vi "asdk Send.vi"(8 "error in (no error)":errorcluster, 10 "value":dbl[](array[numeric]), 11 "pDm":u32) -> (0 "error out":errorcluster, 3 "pDm out":u32)   [LabVIEW 2019, in "ASDK.lvlib"]
doc: "ASDK_API COMPL_STAT asdkSend( asdkDM *pDm, const Scalar *value );"
uses:
  <userlib>/asdk.lib/ASDK.lvlib
  ASDK.dll
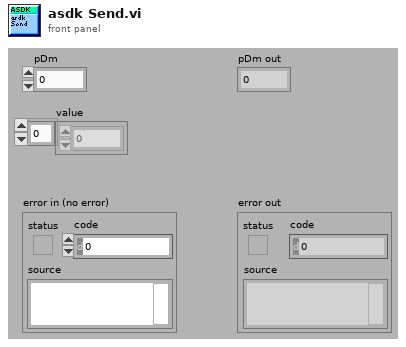
[diagram p1: front panel]
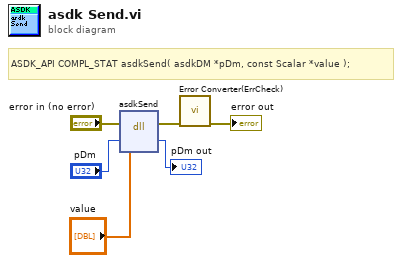
[diagram p0: block diagram]
diagram:
  # "ASDK_API COMPL_STAT asdkSend( asdkDM *pDm, const Scalar *value );"
  n1 = dll-call lib="ASDK.*" fn="asdkSend"(error in="error in (no error)", "pDm"="pDm", "value"="value") -> (error out=w3:errorcluster, "pDm"=→"pDm out":u32)  [unwired: 4 in, 1 out]
  n2 = call <userlib>:"Error Converter(ErrCheck).vi"("error in (no error)"=w3) -> ("error out"=→"error out":errorcluster)  [unwired: 10 in]
